vi "SELECT ITEM COLUMNS.vi"(0 "Inventory Column Selector":T1={"IDENTIFIER"=TRUE, "BYU ICN #"=TRUE, "ITEM"=TRUE, "BUILDING/ROOM"=FALSE, "LOCATION IN ROOM"=FALSE, "MANUAL"=TRUE, "MANUFACTURER"=FALSE, "MODEL #"=FALSE, "SERIAL #"=FALSE, "DATE ACQUIRED"=FALSE, "BYU ID"=TRUE, "FIRST NAME"=TRUE, "LAST NAME"=TRUE, "CHECK OUT LOCATION"=TRUE, "CHECKED OUT DATE"=TRUE, "DUE DATE"=TRUE, "REMINDER COUNT"=TRUE, "MOST RECENT REMINDER DATE"=TRUE, "COMMENTS"=FALSE}, 2 "DATA IN":string[][](array[string]), 3 "Search Database Results":refnum<vi>) -> (7 "DATA OUT":string[][](array[string]), 9 "HEADERS OUT":string[](array[string]))   [LabVIEW 2019]
uses:
  <vilib>/Utility/miscctls.llb/LVRowAndColumnTypeDef.ctl
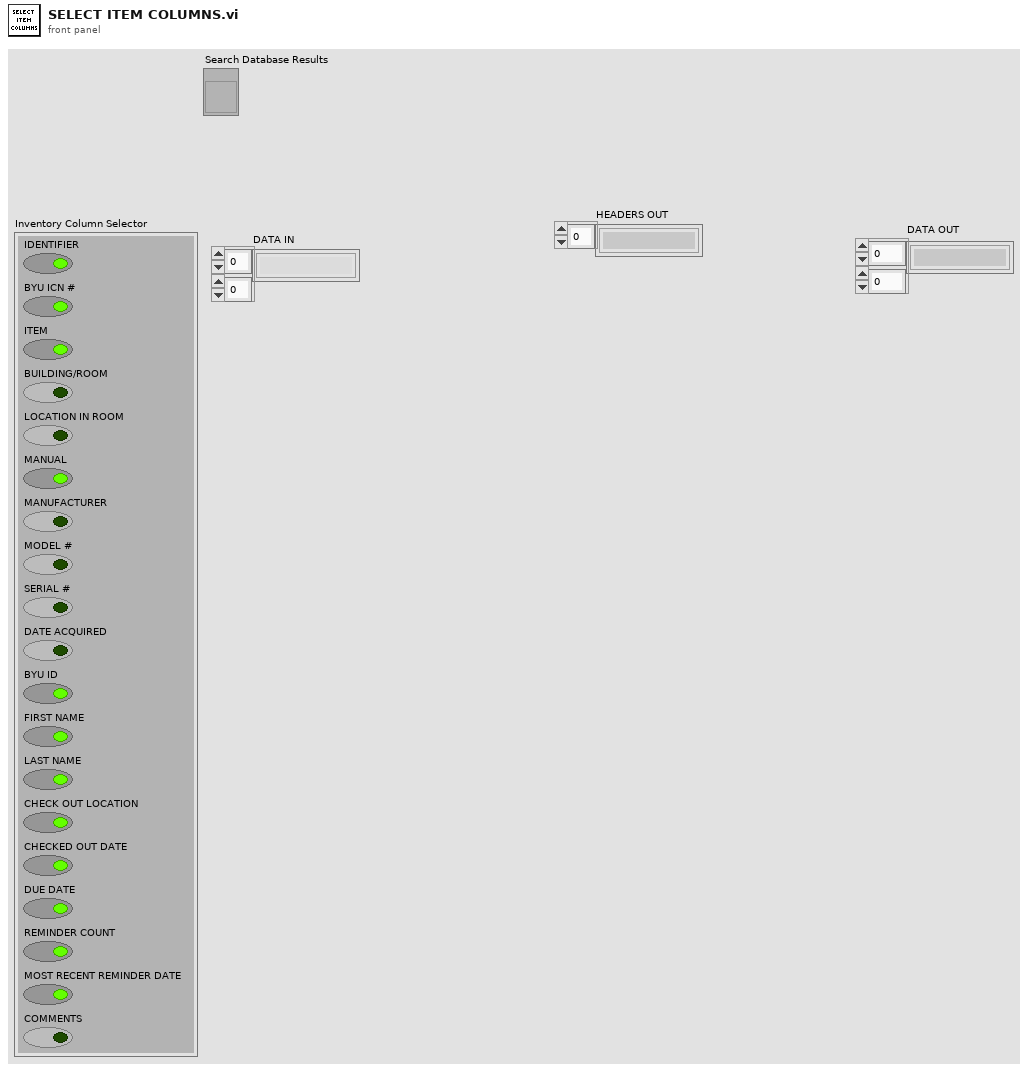
[diagram p1: front panel]
types:
  T1 = cluster{"IDENTIFIER":bool, "BYU ICN #":bool, "ITEM":bool, "BUILDING/ROOM":bool, "LOCATION IN ROOM":bool, "MANUAL":bool, "MANUFACTURER":bool, "MODEL #":bool, "SERIAL #":bool, "DATE ACQUIRED":bool, "BYU ID":bool, "FIRST NAME":bool, "LAST NAME":bool, "CHECK OUT LOCATION":bool, "CHECKED OUT DATE":bool, "DUE DATE":bool, "REMINDER COUNT":bool, "MOST RECENT REMINDER DATE":bool, "COMMENTS":bool}
  T2 = typedef "LVRowAndColumnTypeDef.ctl" = cluster{"Row":i32, "Column":i32}
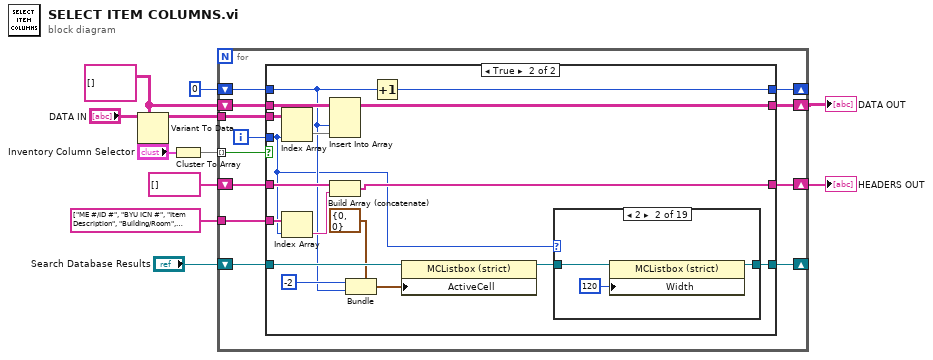
[diagram p0: block diagram]
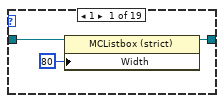
[diagram p3: hidden frame]
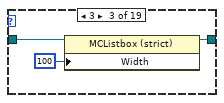
[diagram p4: hidden frame]
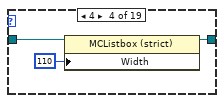
[diagram p5: hidden frame]
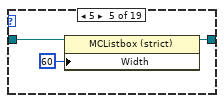
[diagram p6: hidden frame]
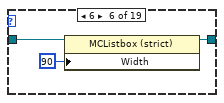
[diagram p7: hidden frame]
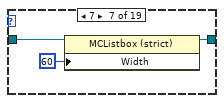
[diagram p8: hidden frame]
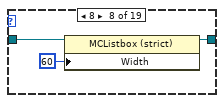
[diagram p9: hidden frame]
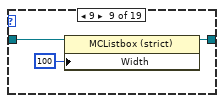
[diagram p10: hidden frame]
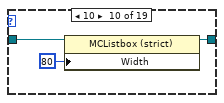
[diagram p11: hidden frame]
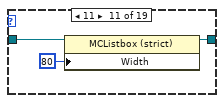
[diagram p12: hidden frame]
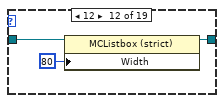
[diagram p13: hidden frame]
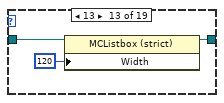
[diagram p14: hidden frame]
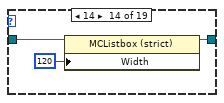
[diagram p15: hidden frame]
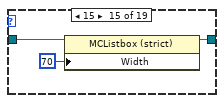
[diagram p16: hidden frame]
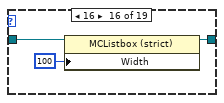
[diagram p17: hidden frame]
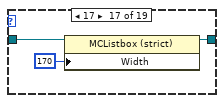
[diagram p18: hidden frame]
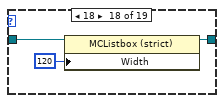
[diagram p19: hidden frame]
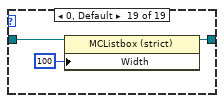
[diagram p20: hidden frame]
diagram:
  w8 = string[][] [] ("DATA OUT")
  n1 = Variant To Data(type=w8, Variant="DATA IN") -> (data=w9:string[][])  [unwired: 1 in, 1 out]
  n2 = Cluster To Array(cluster="Inventory Column Selector") -> (array=w11:bool[])
  n3 = for {
    tunnel: w11 -> [w21] mode=indexing
    tunnel: w9 -> [w23]
    shift-right: [w17] -> w6
    shift-left: w8 -> [w20]
    shift-right: [w18] -> _
    shift-left: 0 -> [w19]
    tunnel: string[] ["ME #/ID #", "BYU ICN #", "Item Description", "Building/Room", "Location In Room", "Manual", "Manufacturer", "Model #", "Serial #", "Date Acquired", "BYU ID #", "First Name", "Last Name", "Check Out Location", "Checked Out Date", "Due Date", "Reminder Count", "Most Recent Reminder Date", "Comments"] ("INVENTORY COLUMN NAMES") -> [w16]
    shift-right: [w14] -> w4
    shift-left: string[] [] ("DATA OUT") -> [w15]
    shift-right: [w12] -> _
    shift-left: "Search Database Results" -> [w13]
    i -> [w22]
    n4 = case shown="True" w21 {
      tunnel: w23 -> [_ w44]
      tunnel: w22 -> [_ w30]
      tunnel: w20 -> [w26 w43]
      tunnel: w19 -> [w27 w31]
      tunnel: [w27 w41] -> w18
      tunnel: [w26 w40] -> w17
      tunnel: w16 -> [_ w39]
      tunnel: w15 -> [w25 w38]
      tunnel: [w25 w36] -> w14
      tunnel: w13 -> [w24 w35]
      tunnel: [w24 w28] -> w12
      frame False {
      }
      frame True {
        n5 = Index Array(array=w44, index (col)=w30) -> (element=w42:string[])  [unwired: 1 in]
        n6 = Index Array(array=w39, index=w30) -> (element=w37:string)
        n7 = Insert Into Array(array=w43, index (col)=w31, new element=w42) -> (w40:string[][])  [unwired: 1 in]
        n8 = Build Array (concatenate)(w38, w37) -> (w36:string[])
        n9 = Bundle(cluster=T2 {"Row"=0, "Column"=0} ("Active Cell:Active Cell"), "Row"=-2, "Column"=w31) -> (w33:T2)
        n10 = Increment(x=w31) -> (x+1=w41:i32)
        n11 = property class="MCListbox (strict)"(reference=w35, "ActiveCell"=w33) -> (reference out=w29:refnum<vi>)  [unwired: 1 in, 1 out]
        n12 = case shown="2" w30 {
          tunnel: w29 -> [w47 w50 w53 w56 w59 w62 w65 w68 w71 w74 w77 w80 w83 w86 w89 w92 w95 w98 w101]
          tunnel: [w45 w48 w51 w54 w57 w60 w63 w66 w69 w72 w75 w78 w81 w84 w87 w90 w93 w96 w99] -> w28
          frame 1 {
            n13 = property class="MCListbox (strict)"(reference=w47, "Width"=u32 80 ("Active Cell:Cell Size:Width")) -> (reference out=w45:refnum<vi>)  [unwired: 1 in, 1 out]
          }
          frame 2 {
            n14 = property class="MCListbox (strict)"(reference=w50, "Width"=u32 120 ("Active Cell:Cell Size:Width")) -> (reference out=w48:refnum<vi>)  [unwired: 1 in, 1 out]
          }
          frame 3 {
            n15 = property class="MCListbox (strict)"(reference=w53, "Width"=u32 100 ("Active Cell:Cell Size:Width")) -> (reference out=w51:refnum<vi>)  [unwired: 1 in, 1 out]
          }
          frame 4 {
            n16 = property class="MCListbox (strict)"(reference=w56, "Width"=u32 110 ("Active Cell:Cell Size:Width")) -> (reference out=w54:refnum<vi>)  [unwired: 1 in, 1 out]
          }
          frame 5 {
            n17 = property class="MCListbox (strict)"(reference=w59, "Width"=u32 60 ("Active Cell:Cell Size:Width")) -> (reference out=w57:refnum<vi>)  [unwired: 1 in, 1 out]
          }
          frame 6 {
            n18 = property class="MCListbox (strict)"(reference=w62, "Width"=u32 90 ("Active Cell:Cell Size:Width")) -> (reference out=w60:refnum<vi>)  [unwired: 1 in, 1 out]
          }
          frame 7 {
            n19 = property class="MCListbox (strict)"(reference=w65, "Width"=u32 60 ("Active Cell:Cell Size:Width")) -> (reference out=w63:refnum<vi>)  [unwired: 1 in, 1 out]
          }
          frame 8 {
            n20 = property class="MCListbox (strict)"(reference=w68, "Width"=u32 60 ("Active Cell:Cell Size:Width")) -> (reference out=w66:refnum<vi>)  [unwired: 1 in, 1 out]
          }
          frame 9 {
            n21 = property class="MCListbox (strict)"(reference=w71, "Width"=u32 100 ("Active Cell:Cell Size:Width")) -> (reference out=w69:refnum<vi>)  [unwired: 1 in, 1 out]
          }
          frame 10 {
            n22 = property class="MCListbox (strict)"(reference=w74, "Width"=u32 80 ("Active Cell:Cell Size:Width")) -> (reference out=w72:refnum<vi>)  [unwired: 1 in, 1 out]
          }
          frame 11 {
            n23 = property class="MCListbox (strict)"(reference=w77, "Width"=u32 80 ("Active Cell:Cell Size:Width")) -> (reference out=w75:refnum<vi>)  [unwired: 1 in, 1 out]
          }
          frame 12 {
            n24 = property class="MCListbox (strict)"(reference=w80, "Width"=u32 80 ("Active Cell:Cell Size:Width")) -> (reference out=w78:refnum<vi>)  [unwired: 1 in, 1 out]
          }
          frame 13 {
            n25 = property class="MCListbox (strict)"(reference=w83, "Width"=u32 120 ("Active Cell:Cell Size:Width")) -> (reference out=w81:refnum<vi>)  [unwired: 1 in, 1 out]
          }
          frame 14 {
            n26 = property class="MCListbox (strict)"(reference=w86, "Width"=u32 120 ("Active Cell:Cell Size:Width")) -> (reference out=w84:refnum<vi>)  [unwired: 1 in, 1 out]
          }
          frame 15 {
            n27 = property class="MCListbox (strict)"(reference=w89, "Width"=u32 70 ("Active Cell:Cell Size:Width")) -> (reference out=w87:refnum<vi>)  [unwired: 1 in, 1 out]
          }
          frame 16 {
            n28 = property class="MCListbox (strict)"(reference=w92, "Width"=u32 100 ("Active Cell:Cell Size:Width")) -> (reference out=w90:refnum<vi>)  [unwired: 1 in, 1 out]
          }
          frame 17 {
            n29 = property class="MCListbox (strict)"(reference=w95, "Width"=u32 170 ("Active Cell:Cell Size:Width")) -> (reference out=w93:refnum<vi>)  [unwired: 1 in, 1 out]
          }
          frame 18 {
            n30 = property class="MCListbox (strict)"(reference=w98, "Width"=u32 120 ("Active Cell:Cell Size:Width")) -> (reference out=w96:refnum<vi>)  [unwired: 1 in, 1 out]
          }
          frame 0, Default {
            n31 = property class="MCListbox (strict)"(reference=w101, "Width"=u32 100 ("Active Cell:Cell Size:Width")) -> (reference out=w99:refnum<vi>)  [unwired: 1 in, 1 out]
          }
        }
      }
    }
  }
  "DATA OUT" <- w6
  "HEADERS OUT" <- w4
